vi "HW File Test.vi"() -> ()   [LabVIEW 2017]
uses:
  Hardware Settings/Hardware Settings.lvclass
  Hardware Settings/Hardware Types/Generic/Type Defs/Owning System.ctl
  Hardware Settings/Hardware Settings.lvclass/Hardware Settings.ctl
  Hardware Settings/Hardware Types/DAQmx/DAQmx.lvclass
  C:/Microcellular Plastics Lab/Hardware Settings/Hardware Types/Generic/Generic Hardware.lvclass
  Hardware Settings/Hardware Types/Generic/Generic Hardware.lvclass/Generic Hardware.ctl
  Hardware Settings/Hardware Types/DAQmx/DAQmx.lvclass/DAQmx.ctl
  Hardware Settings/Hardware Types/Generic/Accessors/Read Owning System.vi
  Hardware Settings/Hardware Types/DAQmx/Accessors/Read DAQmx Task Name.vi
  Hardware Settings/Hardware Types/DAQmx/Accessors/Read Description.vi
  Hardware Settings/Accessors/Read Active Channels.vi
  Hardware Settings/Hardware Types/Generic/Generic Hardware.lvclass
panel:
  out "Array 3":string[](array[string])
  out "Array 2":refnum<k21>[](array[refnum])
  out "Array":T1[](array[typedef])
  out "error out":errorcluster
  out "Hardware Settings.lvclass":refnum<class "Hardware Settings.lvclass">
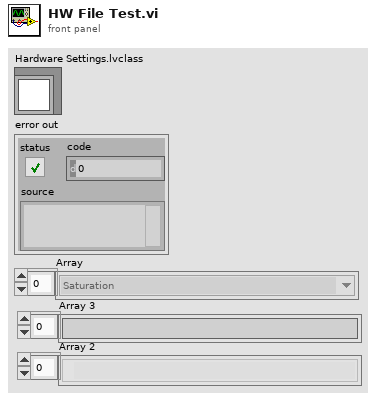
[diagram p1: front panel]
types:
  T1 = typedef "Generic Hardware.lvclass/Owning System.ctl" = enum16{"Saturation", "Expansion"}
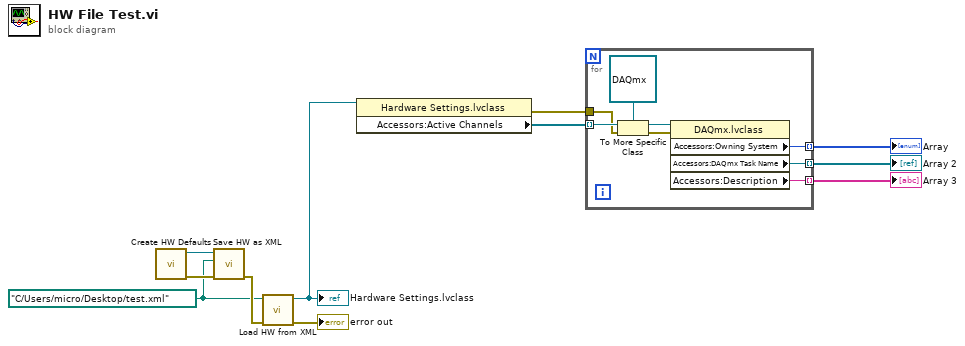
[diagram p0: block diagram]
diagram:
  w8 = path "C:/Users/micro/Desktop/test.xml" ("Path")
  n1 = call "Create HW Defaults.vi"() -> ("error out"=w10:errorcluster, "HW out"=w11:refnum<class "Hardware Settings.lvclass">)  [unwired: 10 in]
  n2 = call "Save HW as XML.vi"("error in (no error)"=w10, "Path"=w8, "Hardware Settings.lvclass"=w11) -> ("error out"=w9:errorcluster)  [unwired: 8 in]
  n3 = call "Load HW from XML.vi"("error in (no error)"=w9, "Path"=w8) -> ("error out"=→"error out":errorcluster, "All Hardware"=w6:refnum<class "Hardware Settings.lvclass">)  [unwired: 8 in]
  "Hardware Settings.lvclass" <- w6
  n4 = property class="Hardware Settings.lvclass"(reference=w6) -> (error out=w1:errorcluster, "Accessors:Active Channels"=w5:refnum<class "Generic Hardware.lvclass">[])  [unwired: 1 in, 1 out]
  n5 = for {
    tunnel: w5 -> [w19] mode=indexing
    tunnel: [w18] -> w4 mode=indexing
    tunnel: [w15] -> w2 mode=indexing
    tunnel: [w14] -> w3 mode=indexing
    tunnel: w1 -> [w13]
    n6 = To More Specific Class(target class=refnum<class "DAQmx.lvclass"> refnum ("DAQmx.lvclass"), reference=w19, error in=w13) -> (specific class reference=w17:refnum<class "DAQmx.lvclass">, error out=w12:errorcluster)
    n7 = property class="DAQmx.lvclass"(reference=w17, error in=w12) -> ("Accessors:Owning System"=w18:T1, "Accessors:DAQmx Task Name"=w15:refnum<k21>, "Accessors:Description"=w14:string)  [unwired: 2 out]
  }
  "Array" <- w4
  "Array 2" <- w2
  "Array 3" <- w3
